vi "Key Pressed.vi"(8 "error in (no error)":errorcluster, 10 "Key Pressed":i32, 11 "Cursor in":refnum<class "Cursor.lvclass">) -> (0 "error out":errorcluster, 3 "Cursor out":refnum<class "Cursor.lvclass">)   [LabVIEW 2020, in "Keypad.lvlib" / "Cursor.lvclass"]
uses:
  Cursor.lvclass
  Keypad/Keypad.lvclass
  Type Def - Cursor Display.ctl
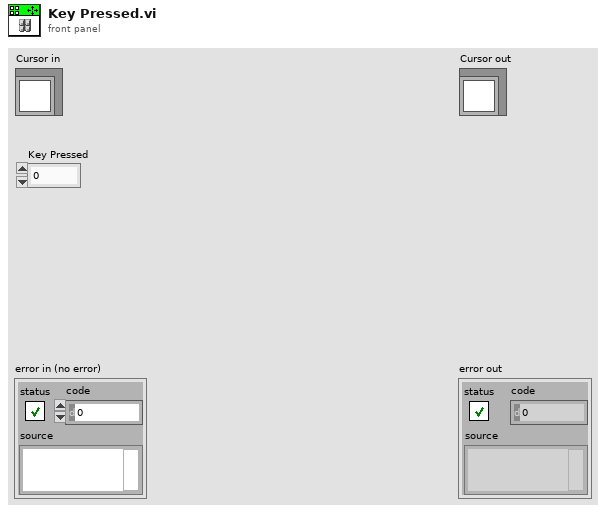
[diagram p1: front panel]
types:
  T1 = typedef "Type Def - Cursor Display.ctl" = cluster{"Up":bool, "Left":bool, "Ctr":bool, "Right":bool, "Down":bool}
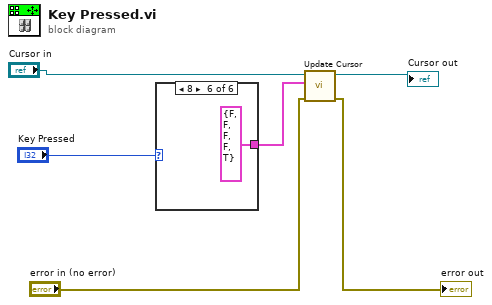
[diagram p0: block diagram]
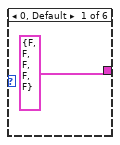
[diagram p2: hidden frame]
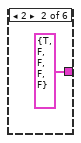
[diagram p3: hidden frame]
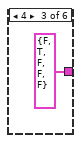
[diagram p4: hidden frame]
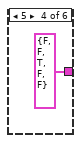
[diagram p5: hidden frame]
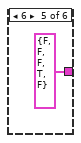
[diagram p6: hidden frame]
diagram:
  n1 = case shown="8" "Key Pressed" {
    tunnel: [T1 {"Up"=FALSE, "Left"=FALSE, "Ctr"=FALSE, "Right"=FALSE, "Down"=FALSE} ("Cursor") T1 {"Up"=TRUE, "Left"=FALSE, "Ctr"=FALSE, "Right"=FALSE, "Down"=FALSE} ("Cursor") T1 {"Up"=FALSE, "Left"=TRUE, "Ctr"=FALSE, "Right"=FALSE, "Down"=FALSE} ("Cursor") T1 {"Up"=FALSE, "Left"=FALSE, "Ctr"=TRUE, "Right"=FALSE, "Down"=FALSE} ("Cursor") T1 {"Up"=FALSE, "Left"=FALSE, "Ctr"=FALSE, "Right"=TRUE, "Down"=FALSE} ("Cursor") T1 {"Up"=FALSE, "Left"=FALSE, "Ctr"=FALSE, "Right"=FALSE, "Down"=TRUE} ("Cursor")] -> w1
    frame 0, Default {
    }
    frame 2 {
    }
    frame 4 {
    }
    frame 5 {
    }
    frame 6 {
    }
    frame 8 {
    }
  }
  n2 = call "Update Cursor.vi"("error in (no error)"="error in (no error)", "Cursor"=w1, "Keypad in"="Cursor in") -> ("error out"=→"error out":errorcluster, "Keypad out"=→"Cursor out":refnum<class "Cursor.lvclass">)  [unwired: 7 in]
